vi "OrdenarPosDefesa.vi"(8 "geometry":T1, 11 "Posições da defesa":dbl[][](array[numeric]) format="%#_13g") -> (3 "Posições ordenadas":dbl[][](array[numeric]) format="%#_13g")   [LabVIEW 2017]
uses:
  Core/Field Size.ctl
  148dee89-422f-4aae-9114-a40a4011e594.vi
  <vilib>/Array/Sort 2D Array - Pop Stack.vi
  <vilib>/Array/Sort 2D Array - Push Stack.vi
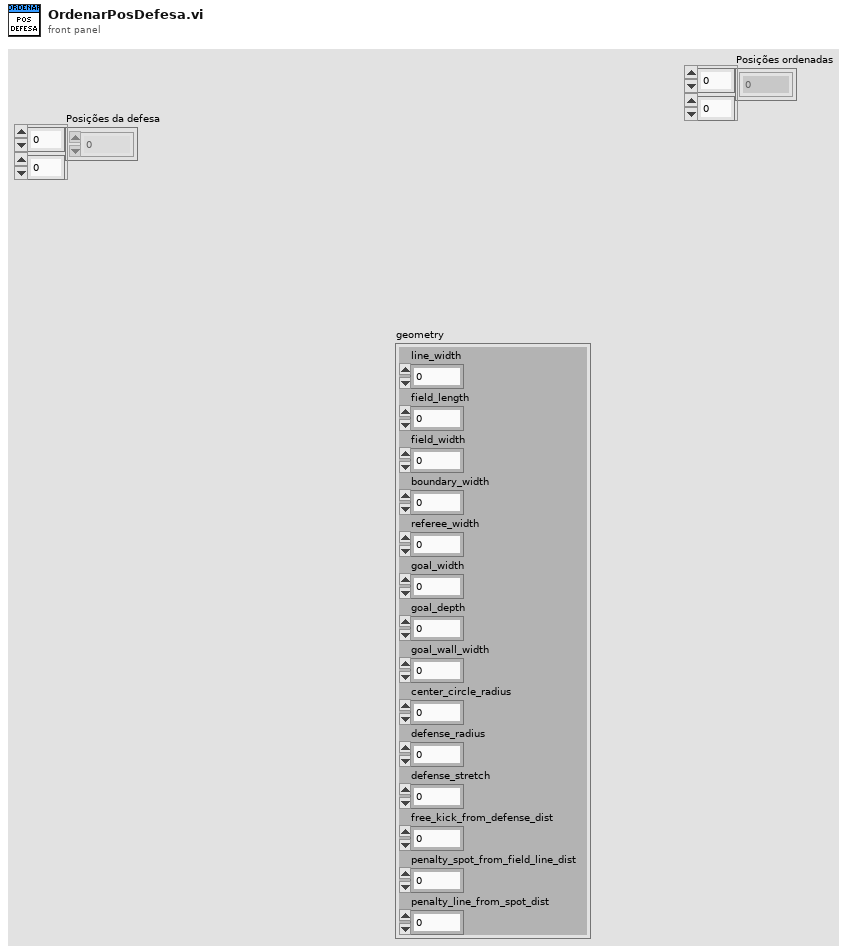
[diagram p1: front panel]
types:
  T1 = typedef "Field Size.ctl" = cluster{"line_width":u32, "field_length":u32, "field_width":u32, "boundary_width":u32, "referee_width":u32, "goal_width":u32, "goal_depth":u32, "goal_wall_width":u32, "center_circle_radius":u32, "defense_radius":u32, "defense_stretch":u32, "free_kick_from_defense_dist":u32, "penalty_spot_from_field_line_dist":u32, "penalty_line_from_spot_dist":u32}
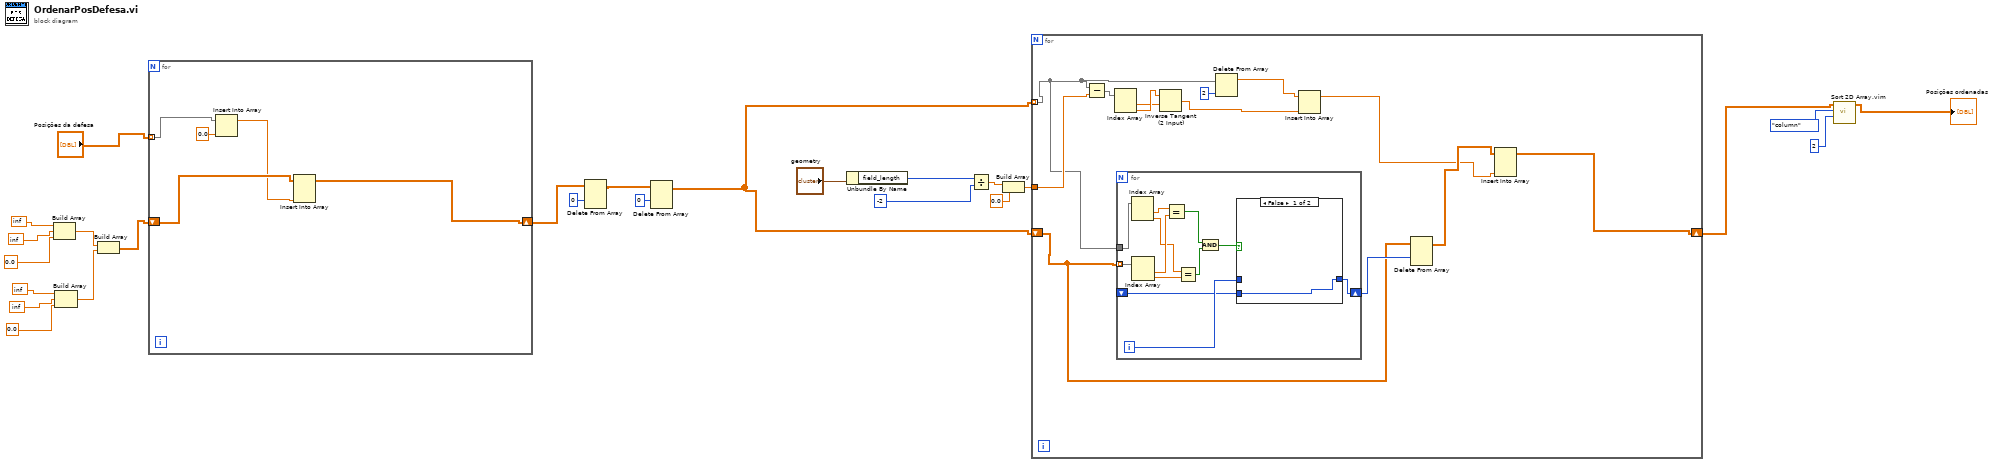
[diagram p0: block diagram]
diagram:
  n1 = Build Array(inf, inf, 0.0) -> (w9:dbl[])
  n2 = Build Array(inf, inf, 0.0) -> (w8:dbl[])
  n3 = Build Array(w9, w8) -> (w7:dbl[][])
  n4 = for {
    tunnel: "Posições da defesa" -> [w30] mode=indexing
    shift-right: [w26] -> w6
    shift-left: w7 -> [w28]
    n5 = Insert Into Array(array=w30, new element=0.0 ("new element/subarray")) -> (w27:dbl[])  [unwired: 1 in]
    n6 = Insert Into Array(array=w28, new element=w27) -> (w26:dbl[][])  [unwired: 2 in]
  }
  n7 = Delete From Array(array=w6, index (row)=0) -> (array with subset deleted=w3:dbl[][])  [unwired: 2 in, 1 out]
  n8 = Delete From Array(array=w3, index (row)=0) -> (array with subset deleted=w2:dbl[][])  [unwired: 2 in, 1 out]
  n9 = Unbundle By Name("geometry") -> ("field_length"=w22:u32)
  n10 = Divide(x=w22, y=-2) -> (x/y=w20:dbl)
  n11 = Build Array(w20, 0.0 ("element")) -> (w18:dbl[])
  n12 = for {
    tunnel: w2 -> [w34] mode=indexing
    shift-right: [w35] -> w17
    shift-left: w2 -> [w38]
    tunnel: w18 -> [w43]
    n13 = Subtract(x=w34, y=w43) -> (x-y=w42:dbl[])
    n14 = Index Array(array=w42) -> (element #1=w40:dbl, element #2=w41:dbl)  [unwired: 2 in]
    n15 = for {
      tunnel: w34 -> [w55]
      tunnel: w38 -> [w54] mode=indexing
      shift-right: [w45] -> w39
      shift-left: _ -> [w44]
      i -> [w46]
      n16 = Index Array(array=w55) -> (element #1=w53:dbl, element #2=w50:dbl)  [unwired: 2 in]
      n17 = Index Array(array=w54) -> (element #1=w52:dbl, element #2=w51:dbl)  [unwired: 2 in]
      n18 = Equal?(x=w53, y=w52) -> (x = y?=w49:bool)
      n19 = Equal?(x=w50, y=w51) -> (x = y?=w48:bool)
      n20 = And(x=w49, y=w48) -> (x .and. y?=w47:bool)
      n21 = case shown="False" w47 {
        tunnel: [w56 w57] -> w45
        tunnel: w46 -> [_ w57]
        tunnel: w44 -> [w56 _]
        frame False {
        }
        frame True {
        }
      }
    }
    n22 = Inverse Tangent (2 Input)(1:w40, 2:w41) -> (0:w31:dbl)
    n23 = Delete From Array(array=w34, index=2) -> (array with subset deleted=w32:dbl[])  [unwired: 1 in, 1 out]
    n24 = Insert Into Array(array=w32, new element=w31) -> (w36:dbl[])  [unwired: 1 in]
    n25 = Delete From Array(array=w38, index (row)=w39) -> (array with subset deleted=w37:dbl[][])  [unwired: 2 in, 1 out]
    n26 = Insert Into Array(array=w37, new element=w36) -> (w35:dbl[][])  [unwired: 2 in]
  }
  n27 = call "Sort 2D Array.vim"("index"=2, "dimension to index (column)"=enum16{"column", "row"}."column", "2D array"=w17) -> ("sorted 2D array"=→"Posições ordenadas":dbl[][])  [unwired: 7 in, 1 out]
